vi "(SubVI)I2C_8Bit-8Bit_Read_Sequential.vi"(5 "Log Ref":refnum<vi>, 7 "Clock":T1=enum."400kHz", 8 "error in (no error)":errorcluster caption="에러 입력(에러 없음)", 9 "Size to Read":u16, 10 "Start Address":u8, 11 "ID":u8) -> (0 "error out":errorcluster caption="에러 출력", 2 "Log":string, 3 "Read Data":u8[](array[numeric]))   [LabVIEW 2020]
uses:
  Controls/(Ctrl)I2C_Clock.ctl
  Controls/(Ctrl)I2C_RW.ctl
  Controls/(Ctrl)I2C_Data Size.ctl
  Serial/Controls/(Ctrl)Serial_Write Read Option.ctl
  Variables/(Var)System Variables.vi
  Serial/Instance VIs/(SubVI)Serial_Write-Read.vi
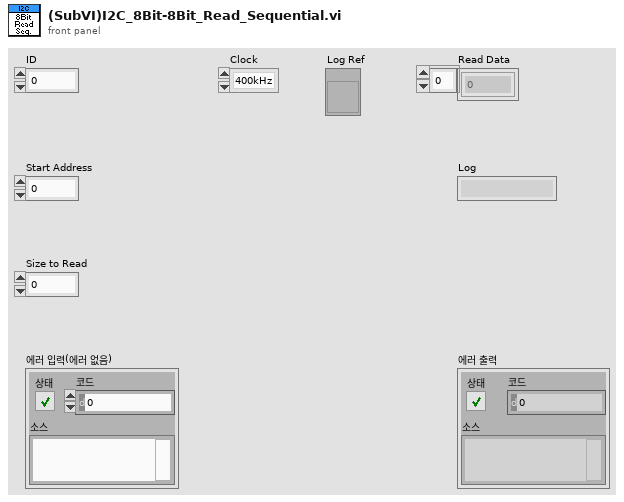
[diagram p1: front panel]
types:
  T1 = typedef "(Ctrl)I2C_Clock.ctl" = enum8{"1MHz", "2MHz", "3MHz", "400kHz"}
  T2 = typedef "(Ctrl)I2C_Data Size.ctl" = enum16{"8Bit_8Bit", "16Bit_16Bit", "16Bit_8Bit"}
  T3 = typedef "(Ctrl)I2C_RW.ctl" = enum16{"Read", "Write"}
  T4 = typedef "(Ctrl)Serial_Write Read Option.ctl" = cluster{"Echo Request":bool, "Header Verification":bool, "Checksum Verification":bool, "User Code Verifiaction":bool}
  T5 = typedef "IC I2C Clock Rate.ctl" = enum8{"50khz", "100khz", "400khz", "1Mhz", "1.2Mhz"}
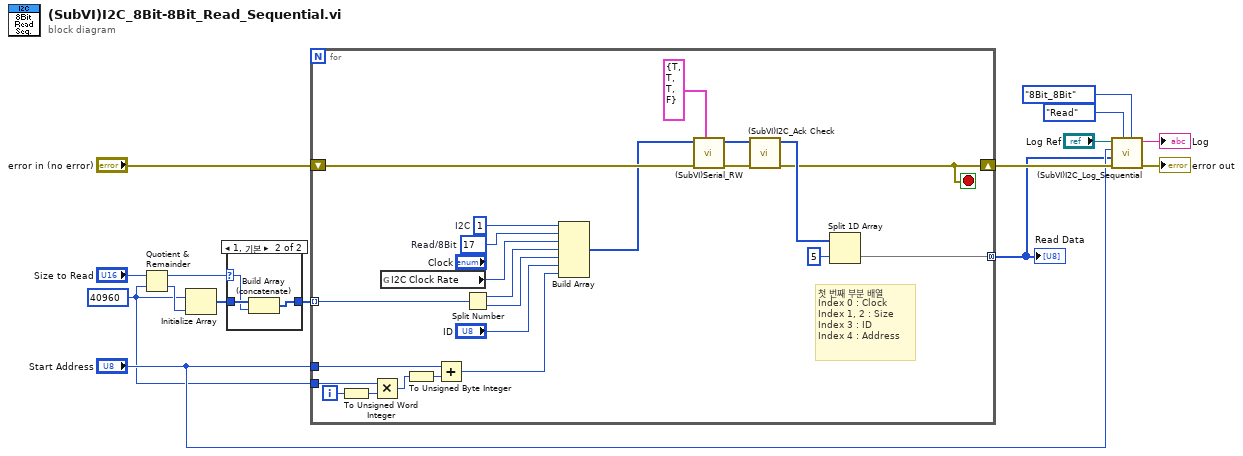
[diagram p0: block diagram]
diagram:
  w2 = u16 40960 ("y")
  n1 = Quotient & Remainder(x="Size to Read", y=w2) -> (x-y*floor(x/y)=w4:u16, floor(x/y)=w6:u16)
  n2 = Initialize Array(w2, w6) -> (w5:u16[])
  n3 = case shown="1, 기본" w4 {
    selector: w4 -> [_ w17]
    tunnel: w5 -> [w16 w19]
    tunnel: [w16 w18] -> w3
    frame 0 {
    }
    frame 1, Default {
      n4 = Build Array (concatenate)(w19, w17) -> (w18:u16[])
    }
  }
  n5 = for {
    tunnel: [w33] -> w1 mode=concatenating
    tunnel: "Start Address" -> [w29]
    tunnel: w3 -> [w28] mode=indexing
    shift-right: [w21] -> w9
    shift-left: "error in (no error)" -> [w42]
    tunnel: w2 -> [w27]
    i -> [w22]
    stop <- w21 stop-if-true
    w40 = u8 17  # Read/8Bit
    w41 = u8 1  # I2C
    # "첫 번째 부분 배열\nIndex 0 : Clock\nIndex 1, 2 : Size\nIndex 3 : ID\nIndex 4 : Address"
    n6 = To Unsigned Word Integer(number=w22) -> (unsigned 16bit integer=w26:u16)
    n7 = Multiply(x=w27, y=w26) -> (x*y=w24:u16)
    n8 = global read "(Var)System Variables.vi" "I2C Clock Rate"() -> (w20:T5)
    n9 = To Unsigned Byte Integer(number=w24) -> (unsigned 8bit integer=w23:u8)
    n10 = Add(x=w29, y=w23) -> (x+y=w25:u8)
    n11 = Split Number(x=w28) -> (hi(x)=w39:u8, lo(x)=w38:u8)
    n12 = Build Array(w41, w40, w20, w39, w38, "ID", w25) -> (w30:u8[])
    n13 = call-poly "(SubVI)Serial_RW.vi"("Option"=T4 {"Echo Request"=TRUE, "Header Verification"=TRUE, "Checksum Verification"=TRUE, "User Code Verifiaction"=FALSE}, "error in (no error)"=w42, "Data to Write"=w30) -> ("error out"=w32:errorcluster, "Read Data"=w34:u8[])  [unwired: 6 in, 1 out]
    n14 = call "(SubVI)I2C_Ack Check.vi"("에러 입력(에러 없음)"=w32, "Read Data"=w34) -> ("에러 출력"=w21:errorcluster, "Read Data Out"=w31:u8[])  [unwired: 8 in]
    n15 = Split 1D Array(array=w31, index=5 ("인덱스")) -> (second subarray=w33:u8[])  [unwired: 1 out]
  }
  "Read Data" <- w1
  n16 = call "(SubVI)I2C_Log_Sequential.vi"("Data Size"=(Ctrl)I2C_Data_Size."8Bit_8Bit", "R/W"=(Ctrl)I2C_RW."Read", "error in (no error)"=w9, "Data Array"=w1, "Start Address"="Start Address", "Log Ref"="Log Ref") -> ("error out"=→"error out":errorcluster, "Log"=→"Log":string)  [unwired: 4 in]
